vi "Send UDP Info to TL.vi"(8 "error in":errorcluster, 10 "UDP Info":T1) -> (0 "error out":errorcluster)   [LabVIEW 2021, in "RT Interpreter.lvlib"]
doc: "_____\nCreated using DQMH Framework: Event Scripter 7.1.2.1547."
uses:
  RT Interpreter.lvlib
  Send UDP Info to TL Argument--cluster.ctl
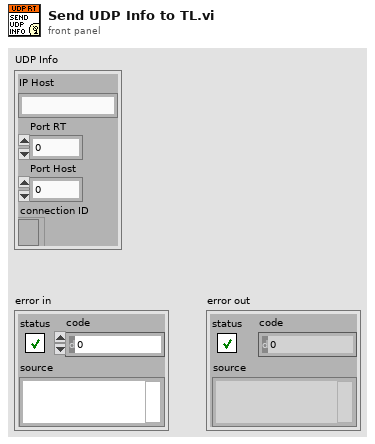
[diagram p1: front panel]
types:
  T1 = cluster{"IP Host":string, "Port RT":u16, "Port Host":u16, "connection ID":refnum<k16>}
  T2 = typedef "RT Interpreter.lvlib/Send UDP Info to TL Argument--cluster.ctl" = cluster{"UDP Info":cluster{"IP Host":string, "Port RT":u16, "Port Host":u16, "connection ID":refnum<k16>}}
  T3 = typedef "RT Interpreter.lvlib/Broadcast Events--cluster.ctl" = cluster{"Module Did Init":refnum<user-event>, "Status Updated":refnum<user-event>, "Error Reported":refnum<user-event>, "Module Did Stop":refnum<user-event>, "Update Module Execution Status":refnum<user-event>, "Send UDP Info to TL":refnum<user-event>}
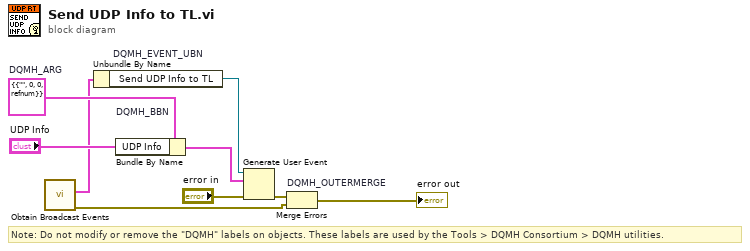
[diagram p0: block diagram]
diagram:
  w4 = T2 {"UDP Info"={"IP Host"="", "Port RT"=0, "Port Host"=0, "connection ID"=refnum}}  # DQMH_ARG
  # "Note: Do not modify or remove the \"DQMH\" labels on objects. These labels are used by the Tools > DQMH Consortium > DQMH utilities."
  n1 = call "Obtain Broadcast Events.vi"() -> ("error out"=w2:errorcluster, "RT Interpreter Broadcast Events"=w1:T3)  [unwired: 10 in]
  n2 = Unbundle By Name "DQMH_EVENT_UBN"(w1) -> ("Send UDP Info to TL"=w6:refnum<user-event>)
  n3 = Bundle By Name "DQMH_BBN"(cluster=w4, "UDP Info"="UDP Info") -> (w7:T2)
  n4 = Generate User Event(user event=w6, event data cluster=w7, error in="error in") -> (error out=w5:errorcluster)  [unwired: 1 in, 1 out]
  n5 = Merge Errors "DQMH_OUTERMERGE"(w5, w2) -> (→"error out":errorcluster)
